vi "CalcPipePoints.vi"(1 "ovalization_data":T2={"AngOval"=[0.0, 60.0, 120.0, 22.5, 45.0, 67.5, 90.0, 112.5, 135.0, 157.5, 180.0], "OvalDiam"=[324.25, 324.6, 324.55, 324.25, 324.55, 324.65, 324.6, 324.65, 324.55, 324.5, 324.4], "Plots"={"Ref"={"X"=[], "Y"=[]}, "Elipse"={"X"=[], "Y"=[]}, "Points"={"X"=[], "Y"=[]}}, "Ampliation"=100.0, "Results"={"MD"=0.0, "mD"=0.0, "Dmed"=0.0, "Oval"=0.0, "ang"=0.0, "X0"=0.0, "Y0"=0.0}, "fit"=[]}) -> (0 "PipePoints":T1)   [LabVIEW 2016]
uses:
  ovalization_data.ctl
  PipePoints.ctl
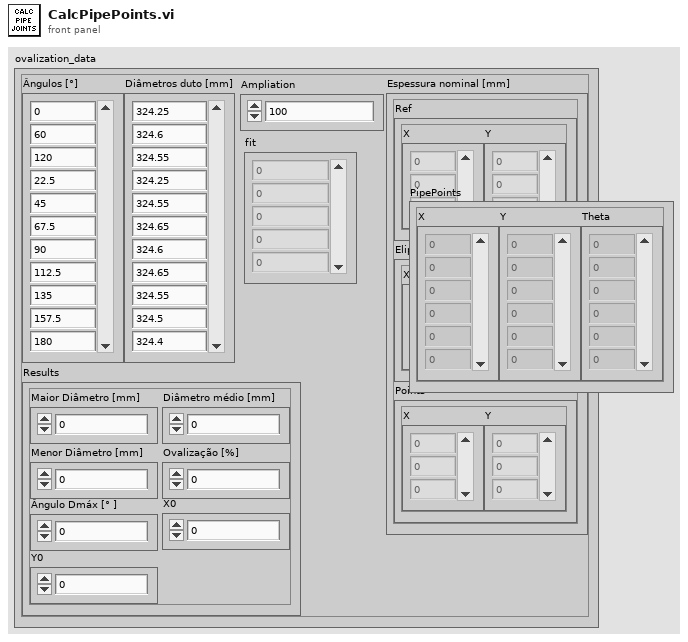
[diagram p1: front panel]
types:
  T1 = typedef "PipePoints.ctl" = cluster{"X":dbl[], "Y":dbl[], "Theta":dbl[]}
  T2 = typedef "ovalization_data.ctl" = cluster{"AngOval":dbl[], "OvalDiam":dbl[], "Plots":cluster{"Ref":cluster{"X":dbl[], "Y":dbl[]}, "Elipse":cluster{"X":dbl[], "Y":dbl[]}, "Points":cluster{"X":dbl[], "Y":dbl[]}}, "Ampliation":dbl, "Results":cluster{"MD":dbl, "mD":dbl, "Dmed":dbl, "Oval":dbl, "ang":dbl, "X0":dbl, "Y0":dbl}, "fit":dbl[]}
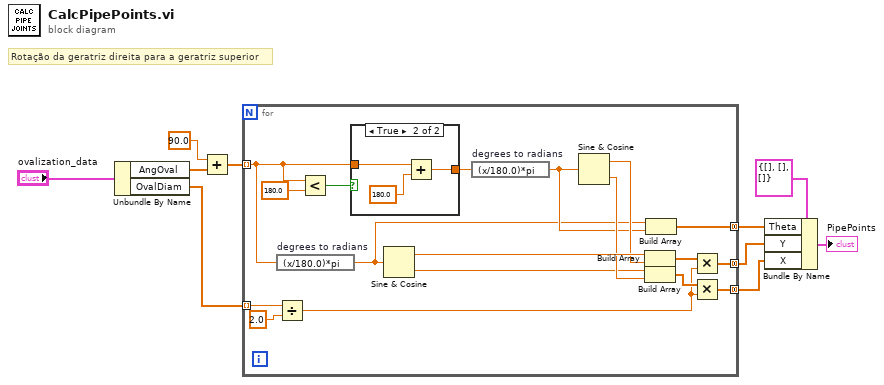
[diagram p0: block diagram]
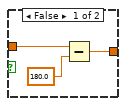
[diagram p2: hidden frame]
diagram:
  # "Rotação da geratriz direita para a geratriz superior"
  n1 = Unbundle By Name("ovalization_data") -> ("AngOval"=w8:dbl[], "OvalDiam"=w6:dbl[])
  n2 = Add(x=90.0 ("y"), y=w8) -> (x+y=w7:dbl[])
  n3 = for {
    tunnel: w6 -> [w28] mode=indexing
    tunnel: w7 -> [w24] mode=indexing
    tunnel: [w15] -> w3 mode=concatenating
    tunnel: [w14] -> w4 mode=concatenating
    tunnel: [w11] -> w2 mode=concatenating
    n4 = expression code="(x/180.0)*pi" "degrees to radians"(w24) -> (w12:dbl)
    n5 = Divide(x=w28, y=2.0) -> (x/y=w16:dbl)
    n6 = Less?(x=w24, y=180.0) -> (x < y?=w25:bool)
    n7 = case shown="True" w25 {
      tunnel: w24 -> [w30 w33]
      tunnel: [w29 w32] -> w23
      frame False {
        n8 = Subtract(x=w30, y=180.0) -> (x-y=w29:dbl)
      }
      frame True {
        n9 = Add(x=w33, y=180.0) -> (x+y=w32:dbl)
      }
    }
    n10 = Sine & Cosine(0:w12) -> (1:w22:dbl, 2:w19:dbl)
    n11 = expression code="(x/180.0)*pi" "degrees to radians"(w23) -> (w13:dbl)
    n12 = Sine & Cosine(0:w13) -> (1:w21:dbl, 2:w20:dbl)
    n13 = Build Array(w22, w21) -> (w18:dbl[])
    n14 = Build Array(w19, w20) -> (w17:dbl[])
    n15 = Build Array(w12, w13) -> (w11:dbl[])
    n16 = Multiply(x=w18, y=w16) -> (x*y=w15:dbl[])
    n17 = Multiply(x=w17, y=w16) -> (x*y=w14:dbl[])
  }
  n18 = Bundle By Name(cluster=T1 {"X"=[], "Y"=[], "Theta"=[]} ("PipePoints"), "Theta"=w2, "Y"=w3, "X"=w4) -> (→"PipePoints":T1)
